vi "CR-字符串检测CCD6.vi"(8 "error in (no error)":errorcluster caption="错误输入（无错误）", 11 "名称或相对路径":string="Template Program") -> (0 "error in (no error) 2":errorcluster caption="错误输入（无错误）")   [LabVIEW 2017]
uses:
  Picture/SaveButtom.ctl
  <vilib>/vision/Pattern Matching.llb/IMAQ Curve Parameters.ctl
  <vilib>/vision/Pattern Matching.llb/IMAQ Match Range Setting.ctl
  Global System.vi
  <vilib>/Utility/xml.llb/Write to XML File(string).vi
panel:
  in  "ROI获取 2":bool
  in  "保存模板位置":bool
  in  "MESS测试按钮":bool
  in  "获取图像":bool
  in  "ROI获取":bool
  in  "创建模板":bool
  in  "保存图像":bool
  out "添加的路径":path
  in  "刷新":bool
  in  "测试按钮":bool
  in  "保存按钮":bool
  in  "Main":enum32{"主参数", "CCD1字符定位参数", "模板匹配参数 ", "测试效果"}(tab)
  in  "字符检测基础参数":T1={"IsNorImage"=TRUE, "Exposure Values"=100289, "ImagePath"=path "C:/Users/hedongpo/Desktop/514-hdp/Alignment Assemble System/Test Picture/B/3.bmp"} caption="参数界面" {"Exposure Values" scale=0.0..200000.0}
  in  "CCD1字符定位参数":T5={"Rectangle"={"Left"=9, "Top"=176, "Right"=891, "Bottom"=836, "Rotation"=0.0}, "Settings"={"Curve Parameters"={"Extraction Mode"=0, "Edge Threshold"=35, "Edge Filter Size"=1, "Min Length"=25, "Row Search Step Size"=15, "Col Search Step Size"=15, "Max Endpoint Gap"=10, "Closed"=FALSE, "Subpixel"=FALSE}, "Match Mode"={"Rotation"=TRUE, "Scale"=FALSE, "Occlusion"=TRUE, "Reserved 1"=FALSE, "Reserved 2"=FALSE, "Reserved 3"=FALSE}, "Range Settings"=[{"Match Constraints"=0, "Min"=-17.0, "Max"=17.0}], "Number of Matches"=1, "Minimum Match Score"=400.0, "SubPixel Accuracy"=FALSE, "Adv. Geometric Match Options 2"=[{"Setup Data Item"=21, "Item Value"=0.0}]}, "Template File Path"=path "D:/Inspect System/Source Code/SubVIs/字符检测VI/aaaa.png"} {"Settings"."Curve Parameters"."Extraction Mode" items=["Normal", "Uniform Regions"]; "Settings"."Curve Parameters"."Edge Filter Size" items=["Fine", "Normal", "Contour Tracing"]; "Settings"."Curve Parameters"."Max Endpoint Gap" min=0; "Settings"."Curve Parameters"."Col Search Step Size" min=1 max=255 step=1; "Settings"."Curve Parameters"."Row Search Step Size" min=1 max=255 step=1; "Settings"."Curve Parameters"."Min Length" min=0; "Settings"."Curve Parameters"."Edge Threshold" min=1 max=350 step=1; "Settings"."Range Settings"."Max" format="%.2f"; "Settings"."Range Settings"."Min" format="%.2f"; "Settings"."Range Settings"."Match Constraints" items=["Rotation Angle (degrees)", "Scale Factor (%)", "Occlusion (%)"]; "Settings"."Adv. Geometric Match Options 2"."Setup Data Item" items=["Curve Extraction Mode", "Curve Edge Threshold", "Curve Edge Filter Size", "Min Curve Length", "Curve Row Search Step Size", "Curve Col Search Step Size", "Curve Max Endpoint Gap", "Extract Closed Curves", "Enable Subpixel Curve Extraction", "Enable Correlation Score", "Enable Subpixel Accuracy", "Subpixel Iterations", "Subpixel Tolerance", "Initial Match List Length", "Enable Target Template Curve Score", "Min Match Separation Distance", "Min Match Separation Angle", "Min Match Separation Scale", "Max Match Overlap", "Enable Coarse Result", "Enable Calibration Support", "Enable Contrast Reversal", "Search Strategy", "Refinement Match Factor", "Subpixel Match Factor"]; "Rectangle"."Rotation" format="%.2f"; "Rectangle"."Left" scale=0.0..1024.0; "Rectangle"."Right" scale=0.0..1024.0}
  in  "字符识别参数":T6={"Parameters (OCR/OCV 1)"={"Threshold Data"={"Method"=enum."Local", "Looking for"=1, "Color Mode"=0, "Kernel Size"={"Width"=32, "Height"=32}, "Ranges"=[{"Min"=1, "Max"=255}]}, "Reject Border"=TRUE, "Number Of Erosions"=0, "Size & Spacing"={"Segment Algorithm"=0, "Min Bounding Rect Width"=1, "Max Bounding Rect Width"=65536, "Min Bounding Rect Height"=1, "Max Bounding Rect Height"=65536, "Min Character Size"=20, "Max Character Size"=65536, "Min Char Spacing"=1, "Max Horiz Element Spacing"=1, "Max Vert Element Spacing"=0, "Max Space Distance"=65536}, "Read Options"={"Read Strategy"=1, "Read Resolution"=2, "Scale Dependant"=FALSE, "Aspect Ratio"=400, "Acceptance Level"=700, "Substitution Character"="?", "MultiLine"=TRUE}, "Valid Characters"=[], "Use Text Pattern"=FALSE, "Orientation"=0, "# Lines Expected"=0, "Number of Blocks"=4}, "Rectangle"={"Left"=0, "Top"=0, "Right"=0, "Bottom"=0, "Rotation"=0.0}, "字符长度判定"=0.0, "Reference System"={"Origin"={"X"=1245.2058, "Y"=1038.7815}, "Angle (deg)"=0.021420227, "Axis Reference"=0}, "File Path (字符库)"=path "D:/Inspect System/Source Code/Template Program/字符模板.abc", "File Path (连接件模板)"=path "D:/Inspect System/Source Code/Template Program/字符检测定位模板.png", "Url"="http://10.6.1.31:8080/MesInnerpackLineIO.asmx", "accessKey"="a45b2d3334ffs_\na45b2d3334ffs_"} {"Reference System"."Axis Reference" items=["Direct", "Indirect"]; "Rectangle"."Rotation" min=-90.0 max=90.0 step=1.0 format="%.2f"; "Rectangle"."Left" scale=0.0..1024.0; "Rectangle"."Right" scale=0.0..1024.0; "Parameters (OCR/OCV 1)"."Threshold Data"."Looking for" items=["Light on Dark", "Dark on Light"]; "Parameters (OCR/OCV 1)"."Threshold Data"."Color Mode" items=["RGB", "HSL", "HSV", "HSI"]; "Parameters (OCR/OCV 1)"."Size & Spacing"."Segment Algorithm" items=["None", "Shortest Segment", "Legacy Auto Split"]; "Parameters (OCR/OCV 1)"."Read Options"."Read Strategy" items=["Aggressive", "Conservative"]; "Parameters (OCR/OCV 1)"."Read Options"."Read Resolution" items=["Low", "Medium", "High"]; "Parameters (OCR/OCV 1)"."Valid Characters"."Pre-defined characters" items=["Any Character", "User-defined Characters", "Alphabetic", "Alphanumeric", "Uppercase Letters", "Lowercase Letters", "Decimal Digits", "Hexadecimal Digits", "Pattern", "Force Space"]; "Parameters (OCR/OCV 1)"."Orientation" items=["Baseline inside", "Baseline outside"]}
  out "原始图像":T7(plugin-control)
  out "ValidateBarcode":string="False,Unable to connect to the remote server"
  out "结果":bool
  out "字符方向判定结果":bool
  out "Data":string
  out "路径输出":path
  in  "Vision Paramter Save Buttom":T8
  out "system time":string
  in  "取消按钮":bool
  # "Range"
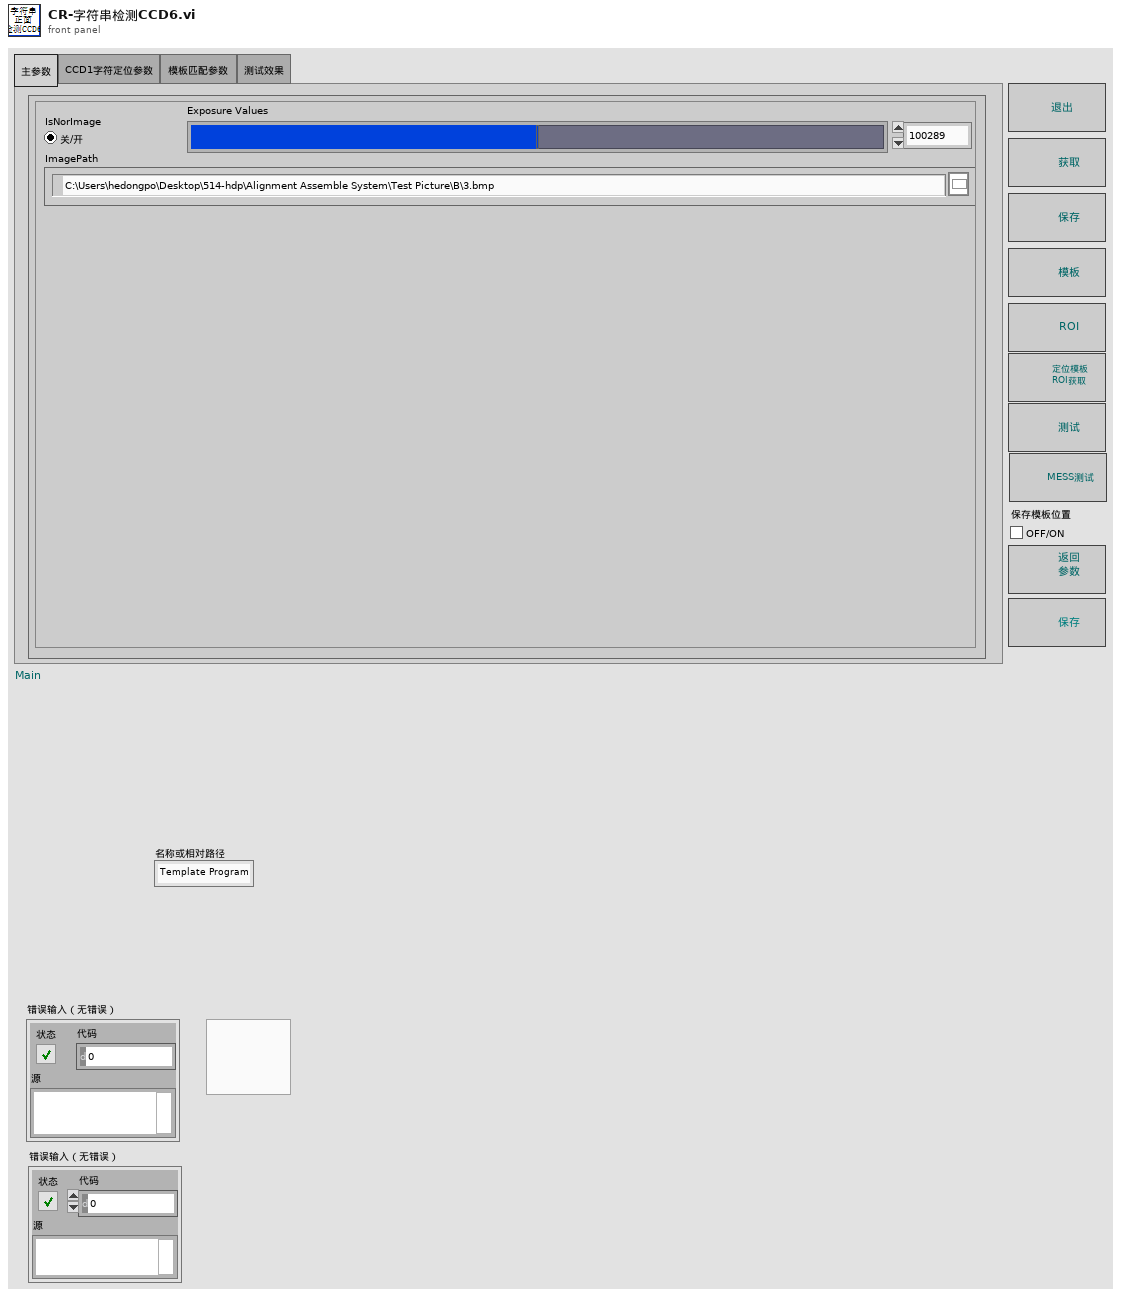
[diagram p1: front panel]
types:
  T1 = cluster{"IsNorImage":bool, "Exposure Values":u32, "ImagePath":path}
  T2 = typedef "IMAQ Rectangle" = cluster{"Left":i32, "Top":i32, "Right":i32, "Bottom":i32, "Rotation":dbl}
  T3 = typedef "IMAQ Curve Parameters.ctl" = cluster{"Extraction Mode":u32, "Edge Threshold":i32, "Edge Filter Size":u32, "Min Length":i32, "Row Search Step Size":i32, "Col Search Step Size":i32, "Max Endpoint Gap":i32, "Closed":bool, "Subpixel":bool}
  T4 = typedef "IMAQ Match Range Setting.ctl" = cluster{"Match Constraints":u32, "Min":dbl, "Max":dbl}
  T5 = cluster{"Rectangle":T2, "Settings":cluster{"Curve Parameters":T3, "Match Mode":cluster{"Rotation":bool, "Scale":bool, "Occlusion":bool, "Reserved 1":bool, "Reserved 2":bool, "Reserved 3":bool}, "Range Settings":T4[], "Number of Matches":i32, "Minimum Match Score":sgl, "SubPixel Accuracy":bool, "Adv. Geometric Match Options 2":cluster{"Setup Data Item":u16, "Item Value":dbl}[]}, "Template File Path":path}
  T6 = cluster{"Parameters (OCR/OCV 1)":cluster{"Threshold Data":cluster{"Method":enum16{"Fixed Range", "Uniform", "Linear", "Non Linear", "Local", "Color"}, "Looking for":u32, "Color Mode":u32, "Kernel Size":cluster{"Width":i32, "Height":i32}, "Ranges":cluster{"Min":i32, "Max":i32}[]}, "Reject Border":bool, "Number Of Erosions":i32, "Size & Spacing":cluster{"Segment Algorithm":u16, "Min Bounding Rect Width":i32, "Max Bounding Rect Width":i32, "Min Bounding Rect Height":i32, "Max Bounding Rect Height":i32, "Min Character Size":i32, "Max Character Size":i32, "Min Char Spacing":i32, "Max Horiz Element Spacing":i32, "Max Vert Element Spacing":i32, "Max Space Distance":i32}, "Read Options":cluster{"Read Strategy":i32, "Read Resolution":i32, "Scale Dependant":bool, "Aspect Ratio":i32, "Acceptance Level":i32, "Substitution Character":string, "MultiLine":bool}, "Valid Characters":cluster{"Pre-defined characters":i32, "User-defined characters":string}[], "Use Text Pattern":bool, "Orientation":u32, "# Lines Expected":u32, "Number of Blocks":i32}, "Rectangle":T2, "字符长度判定":dbl, "Reference System":cluster{"Origin":cluster{"X":sgl, "Y":sgl}, "Angle (deg)":sgl, "Axis Reference":u32}, "File Path (字符库)":path, "File Path (连接件模板)":path, "Url":string, "accessKey":string}
  T7 = typedef "IMAQ Image.ctl" = refnum<image>
  T8 = typedef "SaveButtom.ctl" = bool
  T9 = cluster{"index":i32, "this vi":refnum<vi>, "error out":errorcluster}
  T10 = cluster{"master data":string, "priority":u16, "secondary data":string[]}
  T11 = cluster{"case name":string[], "queue array":refnum<queue>[]}
  T12 = cluster{"Origin":cluster{"X":sgl, "Y":sgl}, "Angle (deg)":sgl, "Axis Reference":u32}
  T13 = typedef "IMAQdx.ctl" = refnum<k21>
  T14 = cluster{"Global Rectangle":i32[], "Contours":cluster{"Contour Type":u32, "ROI Type":u32, "Points":i32[]}[]}
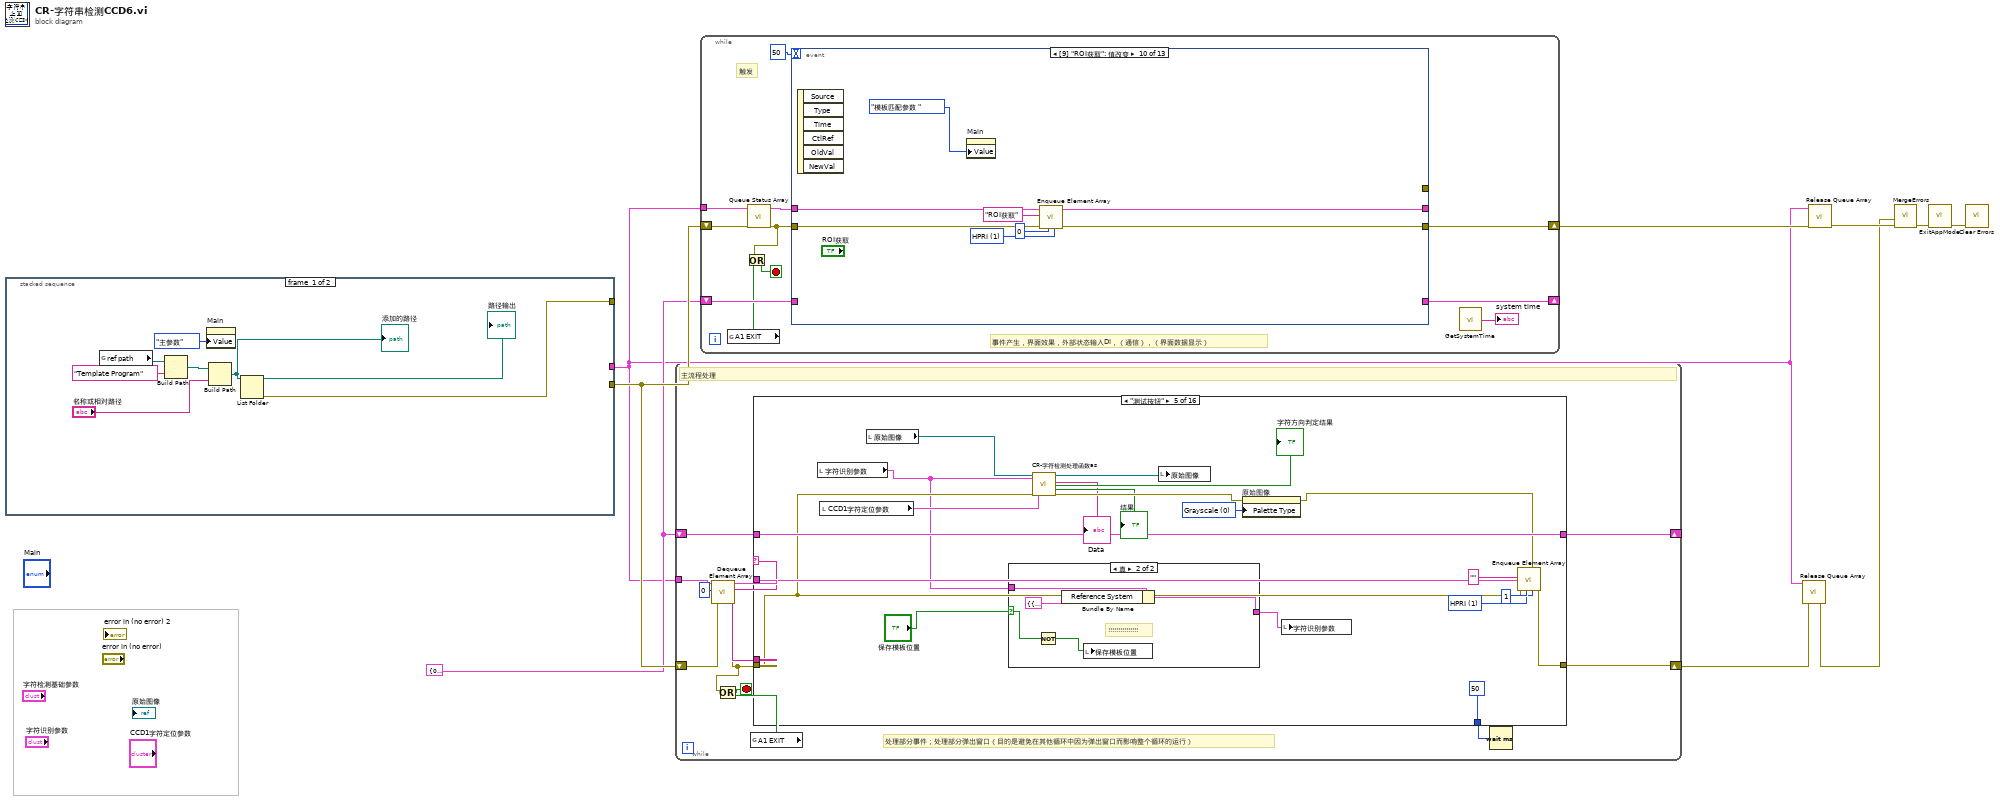
[diagram p0: block diagram]
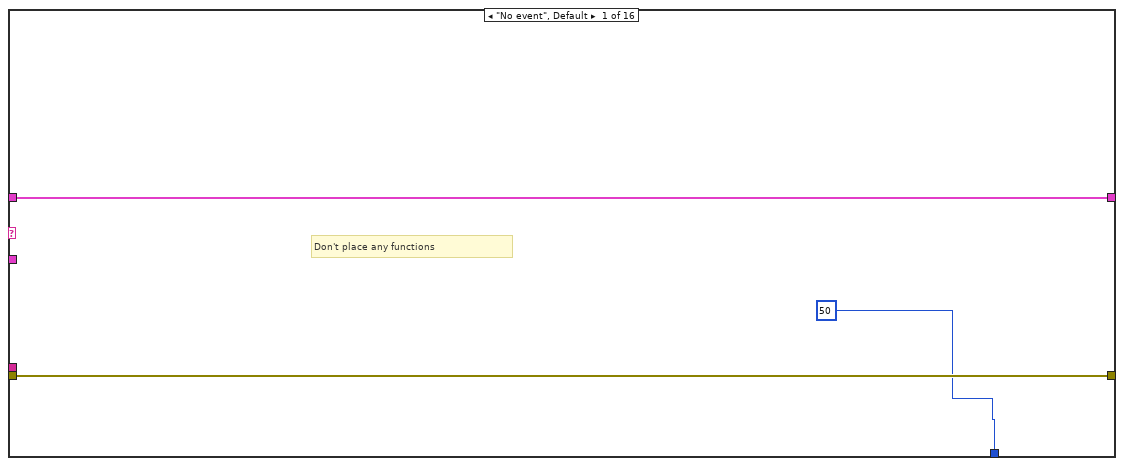
[diagram p2: hidden frame]
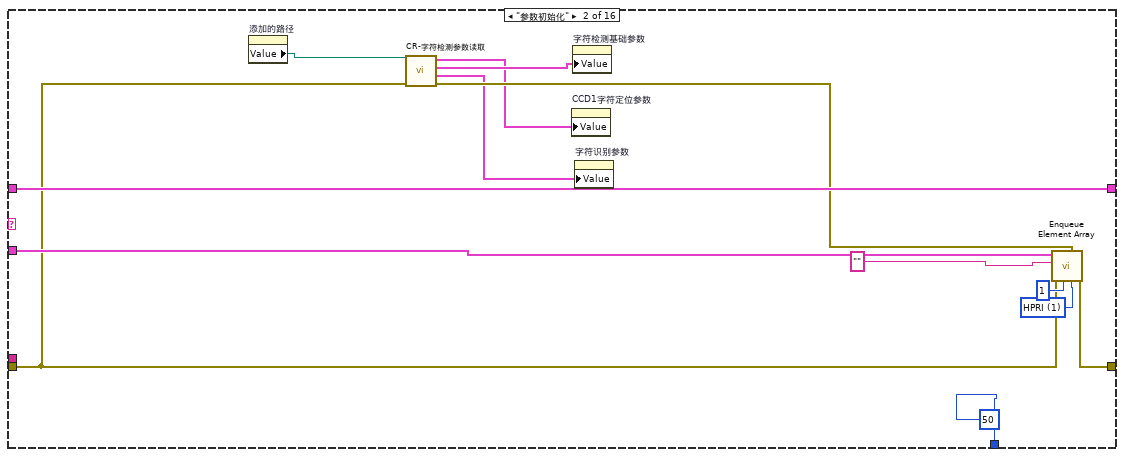
[diagram p3: hidden frame]
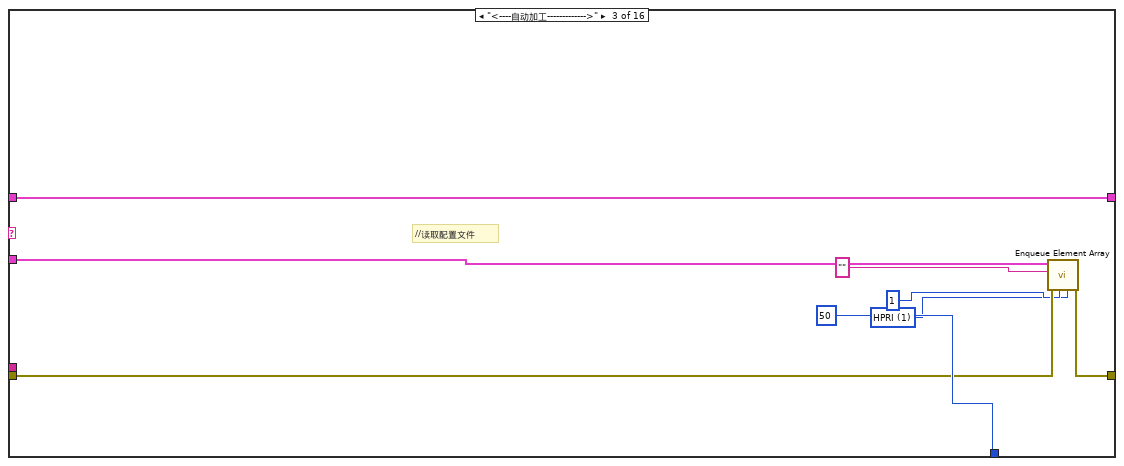
[diagram p4: hidden frame]
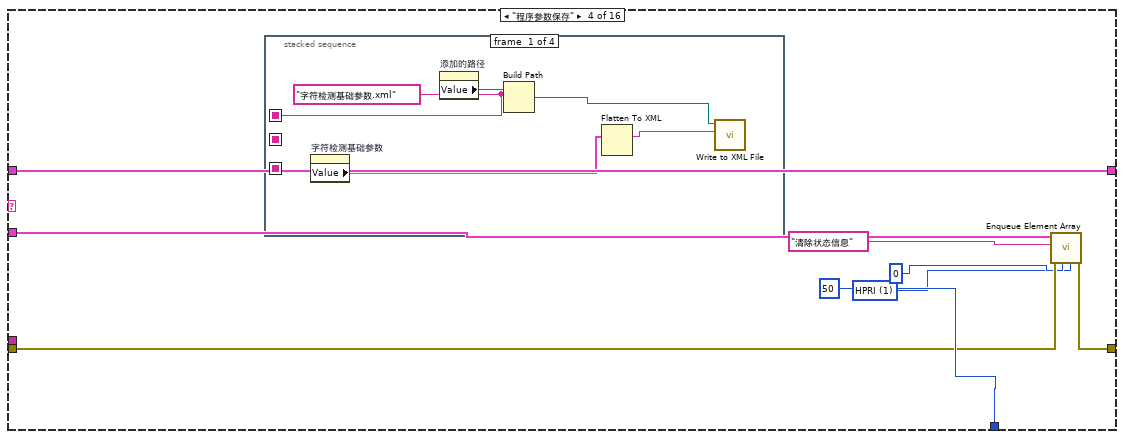
[diagram p5: hidden frame]
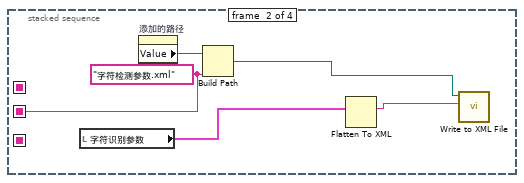
[diagram p6: hidden frame]
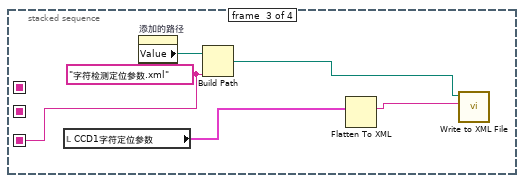
[diagram p7: hidden frame]
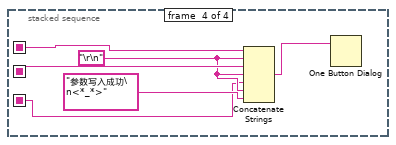
[diagram p8: hidden frame]
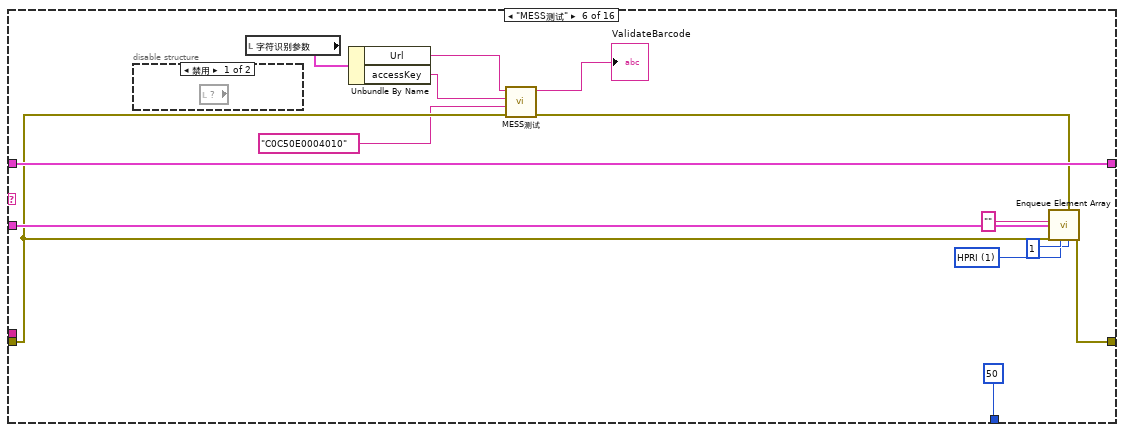
[diagram p10: hidden frame]
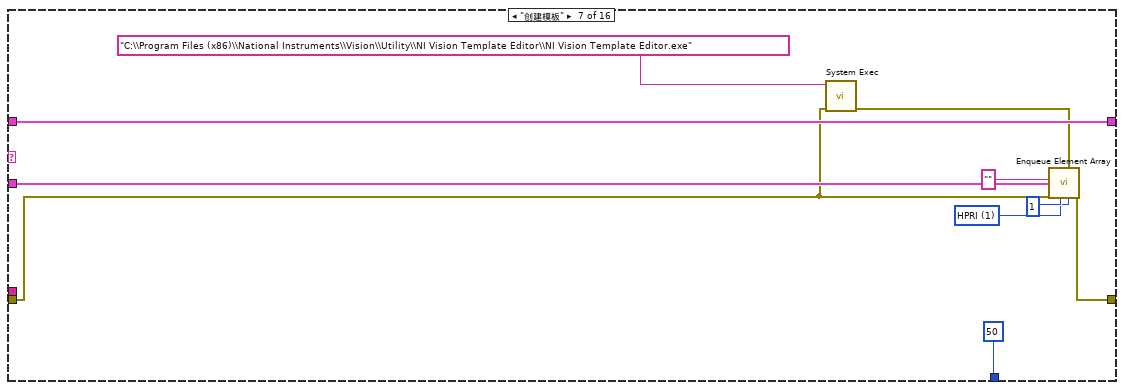
[diagram p12: hidden frame]
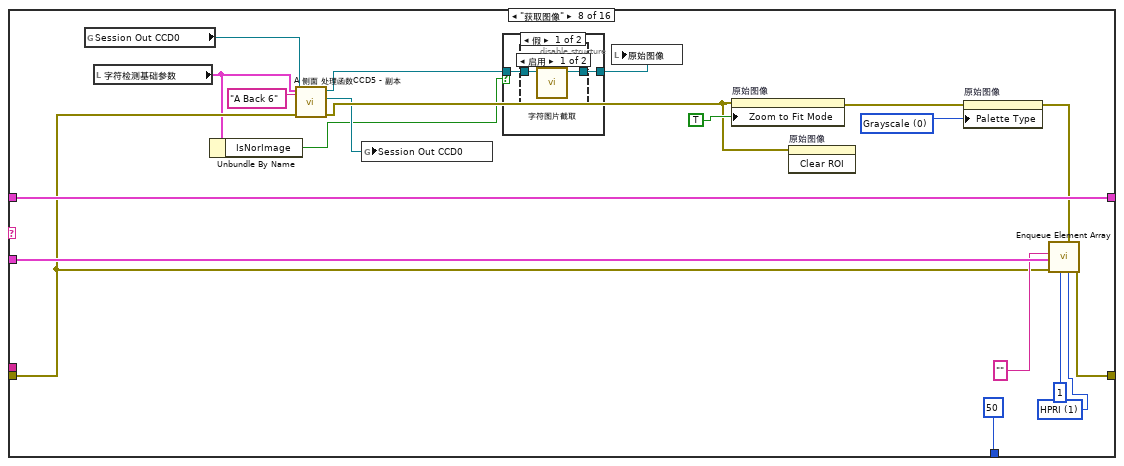
[diagram p13: hidden frame]
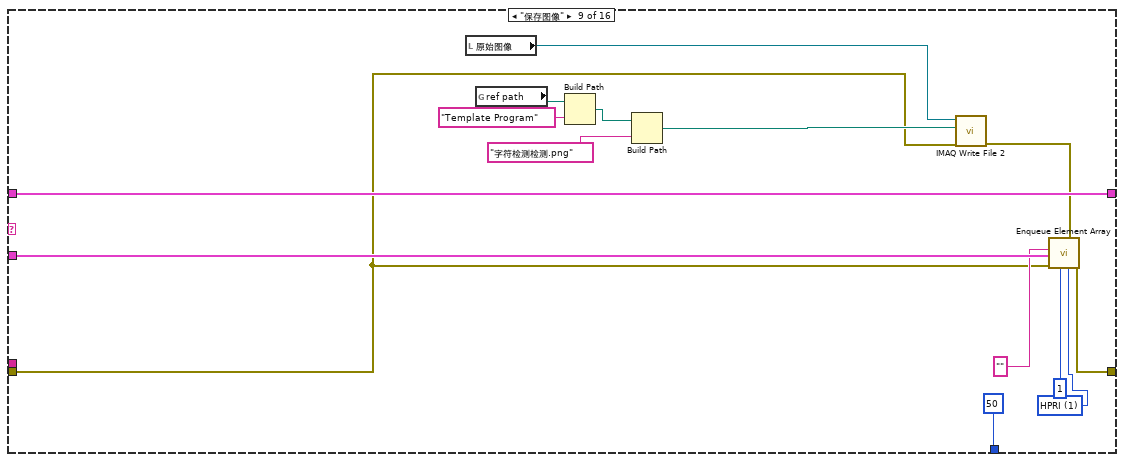
[diagram p16: hidden frame]
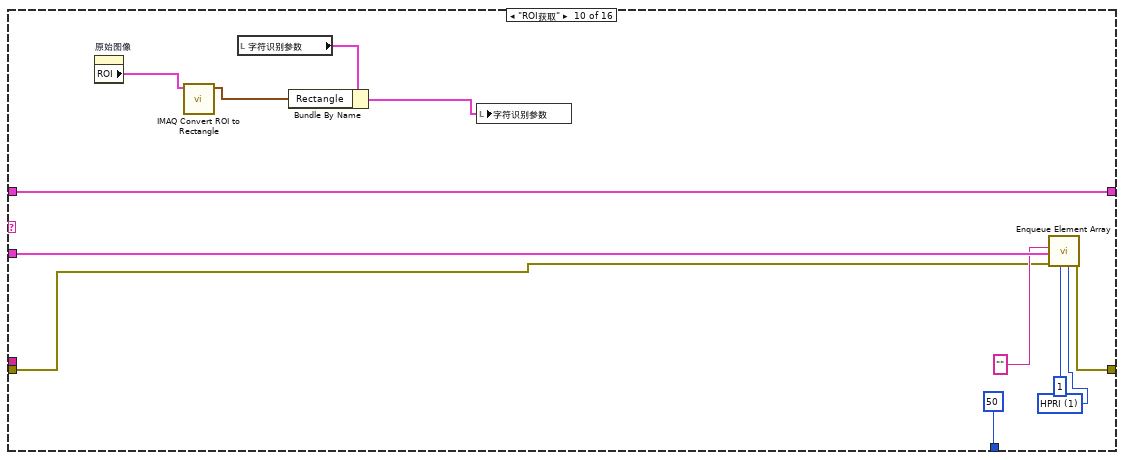
[diagram p17: hidden frame]
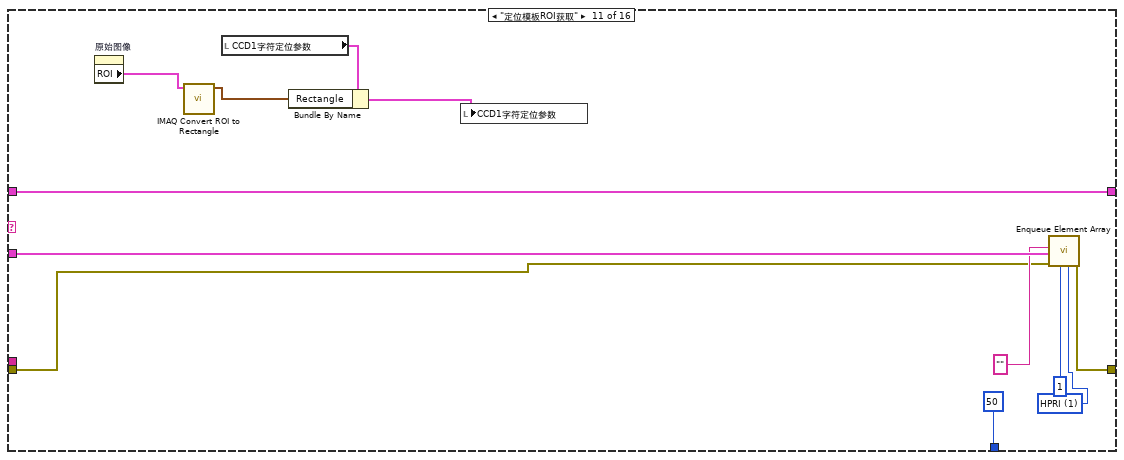
[diagram p18: hidden frame]
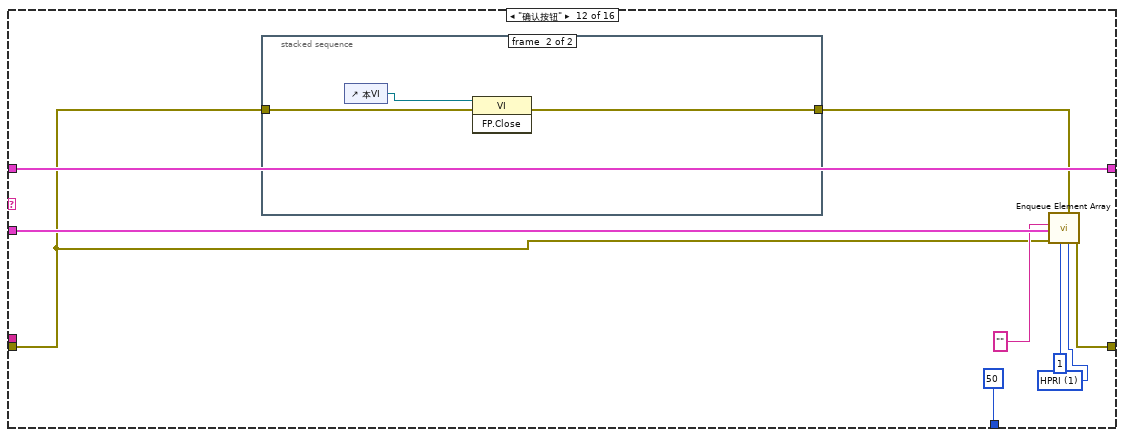
[diagram p19: hidden frame]
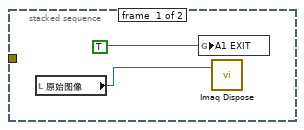
[diagram p20: hidden frame]
diagram:
  w4 = T9 {"index"=0, "this vi"=refnum, "error out"={"status"=FALSE, "code"=0, "source"=""}} ("parameter buffer")
  n1 = stacked-sequence {
    tunnel: [w15 _] -> _
    tunnel: [_ w19] -> w5
    tunnel: [_ w18] -> w1
    frame #0 {
      n2 = global read "Global System.vi" "ref path"() -> (w13:path)
      n3 = Build Path(base path=w13, name or relative path="Template Program" ("名称或相对路径")) -> (appended path=w11:path)
      n4 = property on="Main" class="TabCtl (严格)"("Value"=enum32{"主参数", "CCD1字符定位参数", "模板匹配参数 ", "测试效果"}."主参数" ("Main")) -> ()  [unwired: 2 in, 2 out]
      n5 = Build Path(base path=w11, name or relative path="名称或相对路径") -> (appended path=w17:path)
      "添加的路径" <- w17
      n6 = List Folder(path=w17) -> (path out=→"路径输出":path, error out=w15:errorcluster)  [unwired: 3 in, 2 out]
    }
    frame #1 {
      w27 = string[] ["comm queue1", "data queue 11", "data queue 12", "data queue 13", "data queue 14"]  # queue name
      w28 = 4  # queue num
      w29 = T10 {"master data"="", "priority"=0, "secondary data"=[]}  # element data type
      n7 = call "Obtain Queue Array.vi"("queue name"=w27, "element data type"=w29, "queue num"=w28) -> ("error out"=w23:errorcluster, "queue out"=w24:T11)  [unwired: 2 in, 1 out]
      n8 = call "Enqueue Element Array.vi"("queue index"=0, "error in"=w23, "master data"="参数初始化", "queue in"=w24) -> ("error out"=w22:errorcluster, "queue out"=w21:T11)  [unwired: 6 in]
      n9 = disable-structure shown="启用" {
        disable-tunnel: w22 -> [w35 w36]
        disable-tunnel: w21 -> [w34 w37]
        disable-tunnel: "Loading Variable" ("master data") -> [w33 _]
        disable-tunnel: [w31 w36] -> w19
        disable-tunnel: [w30 w37] -> w18
        frame Disabled {
          n10 = call "Enqueue Element Array.vi"("queue index"=12, "error in"=w35, "master data"=w33, "queue in"=w34) -> ("error out"=w31:errorcluster, "queue out"=w30:T11)  [unwired: 6 in]
        }
        frame Enabled {
        }
      }
    }
  }
  n11 = while {
    shift-right: [w50] -> w3
    shift-left: w5 -> [w41]
    shift-right: [w47] -> _
    shift-left: w4 -> [w48]
    tunnel: w1 -> [w43]
    stop <- w38 stop-if-true
    # "处理部分事件；处理部分弹出窗口（目的是避免在其他循环中因为弹出窗口而影响整个循环的运行）"
    # "主流程处理"
    n12 = call "Dequeue Element Array.vi"("queue in"=w43, "queue index"=0, "error in"=w41) -> ("queue out"=w46:T11, "master data"=w45:string, "secondary data"=w44:string[], "error out"=w40:errorcluster)  [unwired: 2 in, 1 out]
    n13 = global read "Global System.vi" "A1 EXIT"() -> (w39:bool)
    n14 = Or(x=w40, y=w39) -> (x .or. y?=w38:bool)
    n15 = case shown="\"测试按钮\"" w45 {
      tunnel: w46 -> [_ w65 w73 w75 w122 w142 w152 w172 w193 w205 w217 w226 w239 w247 w255 w261]
      tunnel: w40 -> [w52 w58 w69 w79 w111 w136 w145 w165 w181 w199 w211 w220 w235 w243 w251 w258]
      tunnel: [w52 w64 w72 w81 w121 w141 w151 w171 w192 w204 w216 w225 w238 w246 w254 w269] -> w50
      tunnel: [50 50 50 50 50 50 50 50 50 50 50 50 50 50 50 50] -> w49
      tunnel: w48 -> [w53 w60 w70 w76 w117 w137 w147 w167 w188 w200 w212 w221 w236 w244 w252 w267]
      tunnel: [w53 w60 w70 w76 w117 w137 w147 w167 w188 w200 w212 w221 w236 w244 w252 w267] -> w47
      tunnel: w44 -> [_ _ _ _ _ _ _ _ _ _ _ _ _ _ _ _]
      frame "No event", Default {
        # "Don't place any functions"
      }
      frame "参数初始化" {
        w61 = u16 1 items=["HPRI"=1, "LPRI"=0] ("priority")
        n16 = property on="添加的路径" class="Path"() -> ("Value"=w59:path)  [unwired: 2 in, 2 out]
        n17 = call "CR-字符检测参数读取.vi"("error in (no error)"=w58, "基路径"=w59) -> ("error out"=w57:errorcluster, "字符识别参数"=w55:T6, "字符检测基础参数"=w56:T1, "CR-CCD1字符定位参数"=w54:T5)  [unwired: 5 in]
        n18 = property on="CCD1字符定位参数" class="Clust (严格)"("Value"=w54) -> ()  [unwired: 2 in, 2 out]
        n19 = property on="字符检测基础参数" class="Clust (严格)"("Value"=w56) -> ()  [unwired: 2 in, 2 out]
        n20 = property on="字符识别参数" class="Clust (严格)"("Value"=w55) -> ()  [unwired: 2 in, 2 out]
        n21 = call "Enqueue Element Array.vi"("priority"=w61, "device error in"=w57, "queue index"=1, "error in"=w58, "master data"="" ("Element 1"), "queue in"=w65) -> ("error out"=w64:errorcluster)  [unwired: 4 in, 1 out]
      }
      frame "<----自动加工------------->" {
        w67 = u16 1 items=["HPRI"=1, "LPRI"=0] ("priority")
        # "//读取配置文件"
        n22 = call "Enqueue Element Array.vi"("priority"=w67, "queue index"=1, "error in"=w69, "master data"="" ("Element 1"), "queue in"=w73) -> ("error out"=w72:errorcluster)  [unwired: 5 in, 1 out]
      }
      frame "程序参数保存" {
        w77 = u16 1 items=["HPRI"=1, "LPRI"=0] ("priority")
        n23 = stacked-sequence {
          seq-local: [w83 _ _ _] -> [_ _ _ w102]
          seq-local: [_ w92 _ _] -> [_ _ _ w100]
          seq-local: [_ _ w93 _] -> [_ _ _ w98]
          frame #0 {
            w83 = "字符检测基础参数.xml" ("名称或相对路径")
            n24 = property on="字符检测基础参数" class="Clust (严格)"() -> ("Value"=w86:T1)  [unwired: 2 in, 2 out]
            n25 = property on="添加的路径" class="Path"() -> ("Value"=w87:path)  [unwired: 2 in, 2 out]
            n26 = Build Path(base path=w87, name or relative path=w83) -> (appended path=w84:path)
            n27 = Flatten To XML(anything=w86) -> (xml string=w85:string)
            n28 = call-poly <vilib>:"Write to XML File.vi"("XML Input"=w85, "XML File Path"=w84) -> ()  [unwired: 7 in, 3 out]
          }
          frame #1 {
            w92 = "字符检测参数.xml" ("名称或相对路径")
            n29 = local read "字符识别参数"() -> (w88:T6)
            n30 = property on="添加的路径" class="Path"() -> ("Value"=w91:path)  [unwired: 2 in, 2 out]
            n31 = Build Path(base path=w91, name or relative path=w92) -> (appended path=w89:path)
            n32 = Flatten To XML(anything=w88) -> (xml string=w90:string)
            n33 = call-poly <vilib>:"Write to XML File.vi"("XML Input"=w90, "XML File Path"=w89) -> ()  [unwired: 7 in, 3 out]
          }
          frame #2 {
            w93 = "字符检测定位参数.xml" ("名称或相对路径")
            n34 = local read "CCD1字符定位参数"() -> (w94:T5)
            n35 = property on="添加的路径" class="Path"() -> ("Value"=w97:path)  [unwired: 2 in, 2 out]
            n36 = Build Path(base path=w97, name or relative path=w93) -> (appended path=w95:path)
            n37 = Flatten To XML(anything=w94) -> (xml string=w96:string)
            n38 = call-poly <vilib>:"Write to XML File.vi"("XML Input"=w96, "XML File Path"=w95) -> ()  [unwired: 7 in, 3 out]
          }
          frame #3 {
            w99 = "\r\n"
            n39 = Concatenate Strings(w102, w99, w100, w99, w98, w99, "参数写入成功\n<*_*>" ("消息")) -> (w101:string)
            n40 = One Button Dialog(message=w101) -> ()  [unwired: 1 in, 1 out]
          }
        }
        n41 = call "Enqueue Element Array.vi"("priority"=w77, "queue index"=0, "error in"=w79, "master data"="清除状态信息" ("Element 1"), "queue in"=w75) -> ("error out"=w81:errorcluster)  [unwired: 5 in, 1 out]
      }
      frame "测试按钮" {
        w114 = u32 0 items=["Grayscale", "Binary", "Gradient", "Rainbow", "Temperature", "User Defined", "Binary 16 Bit", "Gradient 16 Bit", "Rainbow 16 Bit", "Temperature 16 Bit", "User Defined 16 Bit"] ("Palette:Palette Type")
        w118 = u16 1 items=["HPRI"=1, "LPRI"=0] ("priority")
        n42 = local read "字符识别参数"() -> (w105:T6)
        n43 = local read "CCD1字符定位参数"() -> (w110:T5)
        n44 = local read "原始图像"() -> (w115:T7)
        n45 = case shown="真" "保存模板位置" {
          selector: "保存模板位置" -> [_ w129]
          tunnel: w105 -> [w124 w127]
          tunnel: [w124 w126] -> w108
          frame False {
          }
          frame True {
            # "!!!!!!!!!!!!!!!"
            n46 = Not(x=w129) -> (.not. x?=w128:bool)
            n47 = Bundle By Name(cluster=w127, "Reference System"=T12 {"Origin"={"X"=0.0, "Y"=0.0}, "Angle (deg)"=0.0, "Axis Reference"=0}) -> (w126:T6)
            n48 = local write "保存模板位置"(w128) -> ()
          }
        }
        n49 = call "CR-字符检测处理函数as.vi"("Image in"=w115, "字符识别参数"=w105, "error in (no error)"=w111, "CCD1字符定位参数"=w110) -> ("Image out"=w116:T7, "Data"=→"Data":string, "字符方向判定结果"=→"字符方向判定结果":bool, "结果"=→"结果":bool, "error out"=w113:errorcluster)  [unwired: 10 in, 1 out]
        n50 = local write "原始图像"(w116) -> ()
        n51 = property on="原始图像" class="ImageControl"(error in=w113, "Palette Type"=w114) -> (error out=w112:errorcluster)  [unwired: 1 in, 1 out]
        n52 = local write "字符识别参数"(w108) -> ()
        n53 = call "Enqueue Element Array.vi"("priority"=w118, "device error in"=w112, "queue index"=1, "error in"=w111, "master data"="" ("Element 1"), "queue in"=w122) -> ("error out"=w121:errorcluster)  [unwired: 4 in, 1 out]
      }
      frame "MESS测试" {
        w138 = u16 1 items=["HPRI"=1, "LPRI"=0] ("priority")
        n54 = disable-structure shown="禁用" {
          frame Disabled {
            n55 = local read item#-1() -> ()  [unwired: 1 out]
          }
          frame Enabled {
          }
        }
        n56 = local read "字符识别参数"() -> (w132:T6)
        n57 = Unbundle By Name(w132) -> ("Url"=w131:string, "accessKey"=w130:string)
        n58 = call "MESS测试.vi"("error in (no error)"=w136, "barcode"="C0C50E0004010", "accessKey"=w130, "Url"=w131) -> ("error out"=w135:errorcluster, "ValidateBarcode"=→"ValidateBarcode":string)  [unwired: 6 in]
        n59 = call "Enqueue Element Array.vi"("priority"=w138, "device error in"=w135, "queue index"=1, "error in"=w136, "master data"="" ("Element 1"), "queue in"=w142) -> ("error out"=w141:errorcluster)  [unwired: 4 in, 1 out]
      }
      frame "创建模板" {
        w148 = u16 1 items=["HPRI"=1, "LPRI"=0] ("priority")
        n60 = call <vilib>:"System Exec.vi"("error in (no error)"=w145, "command line"="C:\\Program Files (x86)\\National Instruments\\Vision\\Utility\\NI Vision Template Editor\\NI Vision Template Editor.exe") -> ("error out"=w144:errorcluster)  [unwired: 6 in, 3 out]
        n61 = call "Enqueue Element Array.vi"("priority"=w148, "device error in"=w144, "queue index"=1, "error in"=w145, "master data"="" ("Element 1"), "queue in"=w152) -> ("error out"=w151:errorcluster)  [unwired: 4 in, 1 out]
      }
      frame "获取图像" {
        w162 = u32 0 items=["Grayscale", "Binary", "Gradient", "Rainbow", "Temperature", "User Defined", "Binary 16 Bit", "Gradient 16 Bit", "Rainbow 16 Bit", "Temperature 16 Bit", "User Defined 16 Bit"] ("Palette:Palette Type")
        w168 = u16 1 items=["HPRI"=1, "LPRI"=0] ("priority")
        n62 = global read "Global System.vi" "Session Out CCD0"() -> (w159:T13)
        n63 = local read "字符检测基础参数"() -> (w155:T1)
        n64 = Unbundle By Name(w155) -> ("IsNorImage"=w154:bool)
        n65 = call "A 侧面 处理函数CCD5 - 副本.vi"("Image Name"="A Back 6", "error in (no error)"=w165, "相机选择"=w159, "ParamsUI"=w155) -> ("error out"=w163:errorcluster, "Session Out"=w158:T13, "Image out"=w157:T7)  [unwired: 4 in, 1 out]
        n66 = global write "Global System.vi" "Session Out CCD0"(w158) -> ()
        n67 = case shown="假" w154 {
          tunnel: w157 -> [w175 w179]
          tunnel: [w174 w179] -> w156
          frame False {
            n68 = disable-structure shown="启用" {
              disable-tunnel: w175 -> [w177 w178]
              disable-tunnel: [w176 w178] -> w174
              frame Enabled {
                n69 = call "字符图片截取.vi"("Image"=w177) -> ("Image 3"=w176:T7)  [unwired: 8 in, 2 out]
              }
              frame Disabled {
              }
            }
          }
          frame True {
          }
        }
        n70 = local write "原始图像"(w156) -> ()
        n71 = property on="原始图像" class="ImageControl"(error in=w163, "Zoom to Fit Mode"=TRUE) -> (error out=w161:errorcluster)  [unwired: 1 in, 1 out]
        n72 = invoke on="原始图像" class="ImageControl" method="Clear ROI"(error in=w163) -> ()  [unwired: 2 in, 3 out]
        n73 = property on="原始图像" class="ImageControl"(error in=w161, "Palette Type"=w162) -> (error out=w160:errorcluster)  [unwired: 1 in, 1 out]
        n74 = call "Enqueue Element Array.vi"("priority"=w168, "device error in"=w160, "queue index"=1, "error in"=w165, "master data"="" ("Element 1"), "queue in"=w172) -> ("error out"=w171:errorcluster)  [unwired: 4 in, 1 out]
      }
      frame "保存图像" {
        w189 = u16 1 items=["HPRI"=1, "LPRI"=0] ("priority")
        n75 = local read "原始图像"() -> (w180:T7)
        n76 = global read "Global System.vi" "ref path"() -> (w187:path)
        n77 = Build Path(base path=w187, name or relative path="Template Program" ("名称或相对路径")) -> (appended path=w185:path)
        n78 = Build Path(base path=w185, name or relative path="字符检测检测.png" ("名称或相对路径")) -> (appended path=w183:path)
        n79 = call-poly "IMAQ Write File 2"("error in (no error)"=w181, "File Path"=w183, "Image"=w180) -> ("error out"=w182:errorcluster)  [unwired: 7 in, 1 out]
        n80 = call "Enqueue Element Array.vi"("priority"=w189, "device error in"=w182, "queue index"=1, "error in"=w181, "master data"="" ("Element 1"), "queue in"=w193) -> ("error out"=w192:errorcluster)  [unwired: 4 in, 1 out]
      }
      frame "ROI获取" {
        w201 = u16 1 items=["HPRI"=1, "LPRI"=0] ("priority")
        n81 = property on="原始图像" class="ImageControl"() -> ("ROI"=w198:T14)  [unwired: 2 in, 2 out]
        n82 = call "IMAQ Convert ROI to Rectangle"("ROI Descriptor"=w198) -> ("Rectangle"=w197:T2)  [unwired: 8 in, 1 out]
        n83 = local read "字符识别参数"() -> (w196:T6)
        n84 = Bundle By Name(cluster=w196, "Rectangle"=w197) -> (w195:T6)
        n85 = local write "字符识别参数"(w195) -> ()
        n86 = call "Enqueue Element Array.vi"("priority"=w201, "queue index"=1, "error in"=w199, "master data"="" ("Element 1"), "queue in"=w205) -> ("error out"=w204:errorcluster)  [unwired: 5 in, 1 out]
      }
      frame "定位模板ROI获取" {
        w213 = u16 1 items=["HPRI"=1, "LPRI"=0] ("priority")
        n87 = property on="原始图像" class="ImageControl"() -> ("ROI"=w210:T14)  [unwired: 2 in, 2 out]
        n88 = call "IMAQ Convert ROI to Rectangle"("ROI Descriptor"=w210) -> ("Rectangle"=w209:T2)  [unwired: 8 in, 1 out]
        n89 = local read "CCD1字符定位参数"() -> (w208:T5)
        n90 = Bundle By Name(cluster=w208, "Rectangle"=w209) -> (w207:T5)
        n91 = local write "CCD1字符定位参数"(w207) -> ()
        n92 = call "Enqueue Element Array.vi"("priority"=w213, "queue index"=1, "error in"=w211, "master data"="" ("Element 1"), "queue in"=w217) -> ("error out"=w216:errorcluster)  [unwired: 5 in, 1 out]
      }
      frame "确认按钮" {
        w222 = u16 1 items=["HPRI"=1, "LPRI"=0] ("priority")
        n93 = stacked-sequence {
          tunnel: w220 -> [_ w231]
          tunnel: [_ w230] -> w219
          frame #0 {
            n94 = local read "原始图像"() -> (w228:T7)
            n95 = global write "Global System.vi" "A1 EXIT"(TRUE ("EXIT")) -> ()
            n96 = call "Imaq Dispose"("Image"=w228) -> ()  [unwired: 5 in, 1 out]
          }
          frame #1 {
            n97 = control-ref of="本VI"() -> (w232:refnum<vi>)
            n98 = invoke class="VI" method="FP.Close"(reference=w232, error in=w231) -> (error out=w230:errorcluster)  [unwired: 1 in, 2 out]
          }
        }
        n99 = call "Enqueue Element Array.vi"("priority"=w222, "device error in"=w219, "queue index"=1, "error in"=w220, "master data"="" ("Element 1"), "queue in"=w226) -> ("error out"=w225:errorcluster)  [unwired: 4 in, 1 out]
      }
      frame "<-----自动加工结束--------->" {
        w233 = u16 1 items=["HPRI"=1, "LPRI"=0] ("priority")
        # "//读取配置文件"
        n100 = call "Enqueue Element Array.vi"("priority"=w233, "queue index"=1, "error in"=w235, "master data"="" ("Element 1"), "queue in"=w239) -> ("error out"=w238:errorcluster)  [unwired: 5 in, 1 out]
      }
      frame "<----------手动部分------------->" {
        w241 = u16 1 items=["HPRI"=1, "LPRI"=0] ("priority")
        # "//读取配置文件"
        n101 = call "Enqueue Element Array.vi"("priority"=w241, "queue index"=1, "error in"=w243, "master data"="" ("Element 1"), "queue in"=w247) -> ("error out"=w246:errorcluster)  [unwired: 5 in, 1 out]
      }
      frame "<--------------手动结束---------------->" {
        w249 = u16 1 items=["HPRI"=1, "LPRI"=0] ("priority")
        # "//读取配置文件"
        n102 = call "Enqueue Element Array.vi"("priority"=w249, "queue index"=1, "error in"=w251, "master data"="" ("Element 1"), "queue in"=w255) -> ("error out"=w254:errorcluster)  [unwired: 5 in, 1 out]
      }
      frame "*Emergency alarm" {
        w264 = u16 1 items=["HPRI"=1, "LPRI"=0] ("priority")
        w265 = u16 1 items=["HPRI"=1, "LPRI"=0] ("priority")
        # "发出处理急停信号的命令"
        # "发出处理急停信号的命令"
        n103 = call "Enqueue Element Array.vi"("priority"=w264, "queue index"=0, "error in"=w258, "master data"="" ("Element 1"), "queue in"=w261) -> ("error out"=w259:errorcluster, "queue out"=w260:T11)  [unwired: 5 in]
        n104 = call "SetTestInfoIndex.vi"("test info index"=13) -> ()
        n105 = call "Enqueue Element Array.vi"("priority"=w265, "queue index"=1, "error in"=w259, "master data"="" ("Element 1"), "queue in"=w260) -> ("error out"=w269:errorcluster)  [unwired: 5 in, 1 out]
      }
    }
    n106 = Wait (ms)(milliseconds to wait=w49) -> ()  [unwired: 1 out]
  }
  n107 = while {
    shift-right: [w274] -> w6
    shift-left: w5 -> [w278]
    shift-right: [w276] -> _
    shift-left: w4 -> [w277]
    tunnel: w1 -> [w280]
    stop <- w271 stop-if-true
    # "触发"
    # "事件产生，界面效果，外部状态输入DI，（通信），（界面数据显示）"
    n108 = global read "Global System.vi" "A1 EXIT"() -> (w272:bool)
    n109 = call "Queue Status Array.vi"("error in (no error)"=w278, "queue in"=w280) -> ("error out"=w273:errorcluster, "queue out"=w275:T11)  [unwired: 4 in]
    n110 = Or(x=w273, y=w272) -> (x .or. y?=w271:bool)
    n111 = event shown="[9] \"ROI获取\": 值改变" {
      selector: _ -> [_ _ _ _ _ _ _ _ _ _ _ _ _]
      dyn-events: _ -> [_ _ _ _ _ _ _ _ _ _ _ _ _]
      timeout: 50 -> [_ _ _ _ _ _ _ _ _ _ _ _ _]
      tunnel: w277 -> [w285 w293 _ _ _ _ _ _ _ _ _ _ _]
      tunnel: [w285 w293 _ _ _ _ _ _ _ _ _ _ _] -> w276
      tunnel: [errorcluster {"status"=FALSE, "code"=0, "source"=""} ("error out") _ _ _ _ _ _ _ _ _ _ _ _] -> _
      tunnel: w275 -> [w283 w292 w298 w305 w312 w320 w327 w334 w341 w349 w357 w365 w373]
      tunnel: w273 -> [w282 w291 w297 w304 w311 w319 w326 w333 w340 w348 w356 w364 w372]
      tunnel: [w282 w290 w295 w302 w309 w317 w324 w331 w338 w346 w354 w362 w370] -> w274
      tunnel: [w283 w289 w296 w303 w310 w318 w325 w332 w339 w347 w355 w363 w371] -> _
      event Timeout {
        # "不要在事件结构里面放入\"弹出窗口\"这样的VI保证该循环畅通无阻。"
        n112 = event-data() -> ()  [unwired: 1 in, 1 out]
      }
      event Panel Close? {
        w287 = u16 1 items=["HPRI"=1, "LPRI"=0] ("priority")
        n113 = event-data() -> ()  [unwired: 1 in, 4 out]
        n114 = call "Enqueue Element Array.vi"("priority"=w287, "queue index"=0, "error in"=w291, "master data"="*Exit application", "queue in"=w292) -> ("error out"=w290:errorcluster, "queue out"=w289:T11)  [unwired: 5 in]
        n115 = event-data("Discard?"=TRUE) -> ()  [unwired: 1 in, 1 out]
      }
      event Value Change {
        w300 = u16 1 items=["HPRI"=1, "LPRI"=0] ("priority")
        n116 = event-data() -> ()  [unwired: 1 in, 6 out]
        n117 = call "Enqueue Element Array.vi"("priority"=w300, "queue index"=0, "error in"=w297, "master data"="Vision Paramter Save", "queue in"=w298) -> ("error out"=w295:errorcluster, "queue out"=w296:T11)  [unwired: 5 in]
      }
      event "取消按钮": Value Change {
        w307 = u16 1 items=["HPRI"=1, "LPRI"=0] ("priority")
        n118 = event-data() -> ()  [unwired: 1 in, 6 out]
        n119 = call "Enqueue Element Array.vi"("priority"=w307, "queue index"=0, "error in"=w304, "master data"="确认按钮", "queue in"=w305) -> ("error out"=w302:errorcluster, "queue out"=w303:T11)  [unwired: 5 in]
      }
      event "保存按钮": Value Change {
        w314 = u16 1 items=["HPRI"=1, "LPRI"=0] ("priority")
        n120 = event-data() -> ()  [unwired: 1 in, 6 out]
        n121 = call "Enqueue Element Array.vi"("priority"=w314, "queue index"=0, "error in"=w311, "master data"="程序参数保存", "queue in"=w312) -> ("error out"=w309:errorcluster, "queue out"=w310:T11)  [unwired: 5 in]
      }
      event "获取图像": Value Change {
        w322 = u16 1 items=["HPRI"=1, "LPRI"=0] ("priority")
        n122 = event-data() -> ()  [unwired: 1 in, 6 out]
        n123 = property on="Main" class="TabCtl (严格)"("Value"=enum32{"主参数", "CCD1字符定位参数", "模板匹配参数 ", "测试效果"}."测试效果" ("Main")) -> ()  [unwired: 2 in, 2 out]
        n124 = call "Enqueue Element Array.vi"("priority"=w322, "queue index"=0, "error in"=w319, "master data"="获取图像", "queue in"=w320) -> ("error out"=w317:errorcluster, "queue out"=w318:T11)  [unwired: 5 in]
      }
      event "保存图像": Value Change {
        w329 = u16 1 items=["HPRI"=1, "LPRI"=0] ("priority")
        n125 = event-data() -> ()  [unwired: 1 in, 6 out]
        n126 = call "Enqueue Element Array.vi"("priority"=w329, "queue index"=0, "error in"=w326, "master data"="保存图像", "queue in"=w327) -> ("error out"=w324:errorcluster, "queue out"=w325:T11)  [unwired: 5 in]
      }
      event "创建模板": Value Change {
        w336 = u16 1 items=["HPRI"=1, "LPRI"=0] ("priority")
        n127 = event-data() -> ()  [unwired: 1 in, 6 out]
        n128 = call "Enqueue Element Array.vi"("priority"=w336, "queue index"=0, "error in"=w333, "master data"="创建模板", "queue in"=w334) -> ("error out"=w331:errorcluster, "queue out"=w332:T11)  [unwired: 5 in]
      }
      event "MESS测试按钮": Value Change {
        w343 = u16 1 items=["HPRI"=1, "LPRI"=0] ("priority")
        n129 = event-data() -> ()  [unwired: 1 in, 6 out]
        n130 = call "Enqueue Element Array.vi"("priority"=w343, "queue index"=0, "error in"=w340, "master data"="MESS测试", "queue in"=w341) -> ("error out"=w338:errorcluster, "queue out"=w339:T11)  [unwired: 5 in]
      }
      event "ROI获取": Value Change {
        w351 = u16 1 items=["HPRI"=1, "LPRI"=0] ("priority")
        n131 = event-data() -> ()  [unwired: 1 in, 6 out]
        n132 = property on="Main" class="TabCtl (严格)"("Value"=enum32{"主参数", "CCD1字符定位参数", "模板匹配参数 ", "测试效果"}."模板匹配参数 " ("Main")) -> ()  [unwired: 2 in, 2 out]
        n133 = call "Enqueue Element Array.vi"("priority"=w351, "queue index"=0, "error in"=w348, "master data"="ROI获取", "queue in"=w349) -> ("error out"=w346:errorcluster, "queue out"=w347:T11)  [unwired: 5 in]
      }
      event "ROI获取 2": Value Change {
        w359 = u16 1 items=["HPRI"=1, "LPRI"=0] ("priority")
        n134 = event-data() -> ()  [unwired: 1 in, 6 out]
        n135 = property on="Main" class="TabCtl (严格)"("Value"=enum32{"主参数", "CCD1字符定位参数", "模板匹配参数 ", "测试效果"}."模板匹配参数 " ("Main")) -> ()  [unwired: 2 in, 2 out]
        n136 = call "Enqueue Element Array.vi"("priority"=w359, "queue index"=0, "error in"=w356, "master data"="定位模板ROI获取", "queue in"=w357) -> ("error out"=w354:errorcluster, "queue out"=w355:T11)  [unwired: 5 in]
      }
      event "测试按钮": Value Change {
        w367 = u16 1 items=["HPRI"=1, "LPRI"=0] ("priority")
        n137 = event-data() -> ()  [unwired: 1 in, 6 out]
        n138 = property on="Main" class="TabCtl (严格)"("Value"=enum32{"主参数", "CCD1字符定位参数", "模板匹配参数 ", "测试效果"}."测试效果" ("Main")) -> ()  [unwired: 2 in, 2 out]
        n139 = call "Enqueue Element Array.vi"("priority"=w367, "queue index"=0, "error in"=w364, "master data"="测试按钮", "queue in"=w365) -> ("error out"=w362:errorcluster, "queue out"=w363:T11)  [unwired: 5 in]
      }
      event "刷新": Value Change {
        n140 = event-data() -> ()  [unwired: 1 in, 6 out]
        n141 = disable-structure shown="禁用" {
          disable-tunnel: w373 -> [w377 _]
          disable-tunnel: w372 -> [w376 _]
          disable-tunnel: [w375 _] -> w371
          disable-tunnel: [w374 _] -> w370
          frame Disabled {
            w379 = u16 1 items=["HPRI"=1, "LPRI"=0] ("priority")
            # "刷新"
            n142 = call "Enqueue Element Array.vi"("priority"=w379, "queue index"=0, "error in"=w376, "master data"="刷新", "queue in"=w377) -> ("error out"=w374:errorcluster, "queue out"=w375:T11)  [unwired: 5 in]
          }
          frame Enabled {
          }
        }
        n143 = property on="Main" class="TabCtl (严格)"("Value"=enum32{"主参数", "CCD1字符定位参数", "模板匹配参数 ", "测试效果"}."主参数" ("Main")) -> ()  [unwired: 2 in, 2 out]
      }
    }
    n144 = call "GetSystemTime.vi"() -> ("date/time string"=→"system time":string)  [unwired: 7 in]
  }
  n145 = call "Release Queue Array.vi"("error in"=w3, "queue in"=w1) -> ("error out"=w2:errorcluster)  [unwired: 2 in, 3 out]
  n146 = call "Release Queue Array.vi"("error in"=w6, "queue in"=w1) -> ("error out"=w9:errorcluster)  [unwired: 2 in, 3 out]
  n147 = call "MergeErrors.vi"("error in 3 (no error)"=w2, "error in 4 (no error)"=w9) -> ("error out"=w8:errorcluster)  [unwired: 6 in]
  n148 = call "ExitAppMode.vi"("error in (no error)"=w8) -> ("error out"=w7:errorcluster)  [unwired: 10 in]
  n149 = call <vilib>:"Clear Errors.vi"("error in (no error)"=w7) -> ()  [unwired: 5 in, 2 out]
